vi "SubProperty To Size.vi"(11 "SubProperty":string) -> (3 "Size":T1)   [LabVIEW 2019, in "LSS.lvlib"]
doc: "Parses the subproperty values and converts it to a size with Width and Height.\n\n<b>Inputs</b>\n<b>SubProperty</b> - The value of the subproperrty that will be applied to the control.\n\n<b>Outputs:</b>\n<b>Size</b> - Size cluster containing Width and Height. This can also be used for coordinates."
uses:
  LSS.lvlib
  <vilib>/Utility/miscctls.llb/LVBoundsTypeDef.ctl
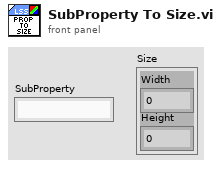
[diagram p1: front panel]
types:
  T1 = typedef "LVBoundsTypeDef.ctl" = cluster{"Width":u32, "Height":u32}
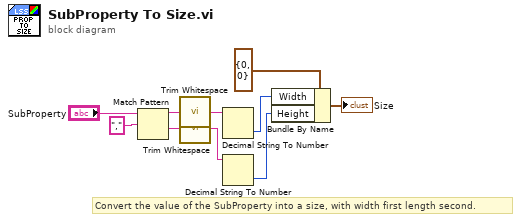
[diagram p0: block diagram]
diagram:
  # "Convert the value of the SubProperty into a size, with width first length second."
  n1 = Match Pattern(string="SubProperty", regular expression=",") -> (before substring=w7:string, after substring=w5:string)  [unwired: 1 in, 2 out]
  n2 = call <vilib>:"Trim Whitespace.vi"("string"=w7) -> ("trimmed string"=w2:string)  [unwired: 1 in]
  n3 = call <vilib>:"Trim Whitespace.vi"("string"=w5) -> ("trimmed string"=w1:string)  [unwired: 1 in]
  n4 = Decimal String To Number(string=w2) -> (number=w6:i32)  [unwired: 2 in, 1 out]
  n5 = Decimal String To Number(string=w1) -> (number=w4:i32)  [unwired: 2 in, 1 out]
  n6 = Bundle By Name(cluster=T1 {"Width"=0, "Height"=0} ("Size"), "Width"=w6, "Height"=w4) -> (→"Size":T1)
